vi "Configure Parameters.vi"(0 "instrument handle":refnum<k15>, 1 "TriggerSource (Immediate)":i32(ring) items=["Immediate"=0, "Video"=1, "AC Line"=2, "External1"=3, "External2"=4, "RF Burst"=5, "Frame"=8, "LXI Lan Event"=10, "LXI Alarm Trigger"=11, "IF"=6, "IQ Magnitude"=7, "DemodulatedI Voltage"=9, "DemodulatedQ Voltage"=12, "IADC Volatge"=13, "QADC Voltage"=14, "AuxiliaryIQ Magnitude"=15, "Software"=16], 2 "TriggerOffset":dbl, 5 "PeakMeasurementEnabled (Off)":bool, 7 "RMSMeasurementEnabled (Off)":bool, 9 "AveragingMeasurementEnabled (Off)":bool, 11 "error in (no error)":errorcluster {"code" format="%.0x"}, 12 "TriggerSlope (Positive)":i32(ring) items=["Positive", "Negative"], 13 "GateLength":dbl) -> (4 "instrument handle out":refnum<k15>, 15 "error out":errorcluster {"code" format="%.0x"})   [LabVIEW 2009, in "Keysight XSAn.lvlib"]
doc: "Sets parameters to the entire list.\n\nSupported Models: M9290A, N8973B, N8974B, N8975B, N8976B, N9000A, N9000B, N9010A, N9010B, N9020A, N9020B, N9030A, N9030B, N9038A, N9040B, N9041B, SPN9003A, SPN9026A"
uses:
  <instrlib>/Keysight XSAn/Keysight XSAn.lvlib
  AgXSAn.dll
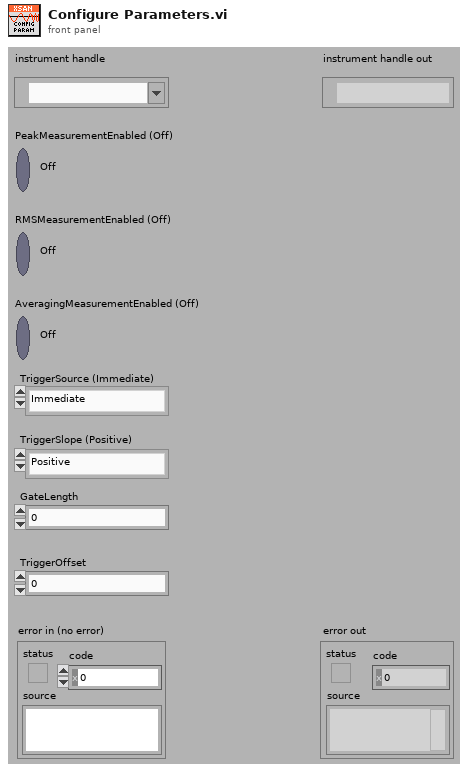
[diagram p1: front panel]
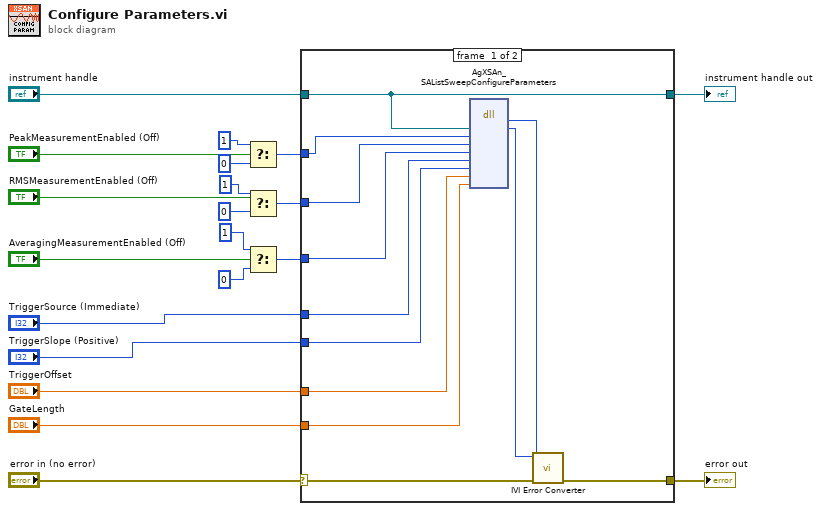
[diagram p0: block diagram]
diagram:
  n1 = Select(t=u16 1, s="PeakMeasurementEnabled (Off)", f=u16 0) -> (s? t:f=w14:u16)
  n2 = Select(t=u16 1, s="RMSMeasurementEnabled (Off)", f=u16 0) -> (s? t:f=w10:u16)
  n3 = Select(t=u16 1, s="AveragingMeasurementEnabled (Off)", f=u16 0) -> (s? t:f=w6:u16)
  n4 = case shown="No Error" "error in (no error)" {
    selector: "error in (no error)" -> [w30 w34]
    tunnel: [w29 w34] -> w20
    tunnel: "instrument handle" -> [w21 w33]
    tunnel: w14 -> [w28 _]
    tunnel: w10 -> [w27 _]
    tunnel: w6 -> [w26 _]
    tunnel: "TriggerSource (Immediate)" -> [w25 _]
    tunnel: "TriggerSlope (Positive)" -> [w24 _]
    tunnel: "TriggerOffset" -> [w23 _]
    tunnel: "GateLength" -> [w22 _]
    tunnel: [w21 w33] -> w1
    frame #0 {
      n5 = dll-call lib="AgXSAn**.dll" fn="AgXSAn_SAListSweepConfigureParameters"("Vi"=w21, "PeakMeasurementEnabled"=w28, "RMSMeasurementEnabled"=w27, "AveragingMeasurementEnabled"=w26, "TriggerSource"=w25, "TriggerSlope"=w24, "TriggerOffset"=w23, "GateLength"=w22) -> (w31:i32, "Vi"=w32:u32)  [unwired: 10 in, 2 out]
      n6 = call <instrlib>:"IVI Error Converter.vi"("error in (no error)"=w30, "IVI error code (0)"=w31, "instrument handle"=w32) -> ("error out"=w29:errorcluster)  [unwired: 7 in, 1 out]
    }
    frame #1 {
    }
  }
  "error out" <- w20
  "instrument handle out" <- w1
